vi "Main Page.vi"(8 "error in (no error)":errorcluster, 11 "Node Ptr":T1 format="%.0x") -> (0 "error out":errorcluster)   [LabVIEW 2015, in "Fuel Injector Analysis Addon System Explorer.lvlib"]
uses:
  Fuel Injector Analysis Addon System Explorer.lvlib
  <vilib>/NI Veristand/Custom Device API/Custom Device Item Ref.ctl
  <vilib>/NI/NI VeriStand Hardware Discovery/Types/Filter Type.ctl
  Shared/Constants.vi
  <vilib>/NI Veristand/Custom Device API/Set Item Property (String).vi
  <vilib>/NI Veristand/Custom Device API/Custom Device API.lvlib
  Shared/Fuel Injector Analysis Addon Shared.lvlib
  <vilib>/NI/NI VeriStand Hardware Discovery/NIVS Hardware Discovery.lvlib
panel:
  in  "RIO Browse":bool
  in  "SHDocVw.IWebBrowser":refnum<k7>(container)
  in  "Description":string
  in  "Sample Rate (Hz)":u32
  in  "RIO Device":string
  in  "Local Bitfile path":path
  in  "Header":cluster{"Section Name":string}={"Section Name"="Custom Device Item Settings"}
  in  "Name":string
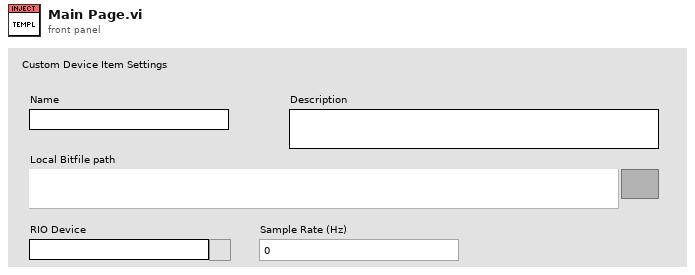
[diagram p1: front panel]
types:
  T1 = typedef "Custom Device API.lvlib/Custom Device Item Ref.ctl" = u64
  T2 = typedef "Custom Device API.lvlib/Custom Device Item Info.ctl" = cluster{"Name":string, "Is Channel":bool, "GUID":string, "Is Waveform":bool}
  T3 = typedef "Fuel Injector Analysis Addon Shared.lvlib/Main Settings.ctl" = cluster{"RIO Device Address":string, "Local bitfile path":path, "RT bitfile path":path, "Number of injectors":u16, "Sample rate (S/s)":u32}
  T4 = typedef "NIVS Hardware Discovery.lvlib/Filter Type.ctl" = enum16{"Device Category", "Product Name", "Ethernet", "XNET", "VISA", "FPGA", "EtherCAT Master", "DAQmx", "GPIB", "Serial"}
  T5 = enum16{"0", "1", "2", "3", "4", "5", "6", "7", "8"}
  T6 = typedef "Custom Device API.lvlib/Custom Device Commands.ctl" = enum16{"Default", "Item renamed", "Shutdown", "Dynamic button pressed"}
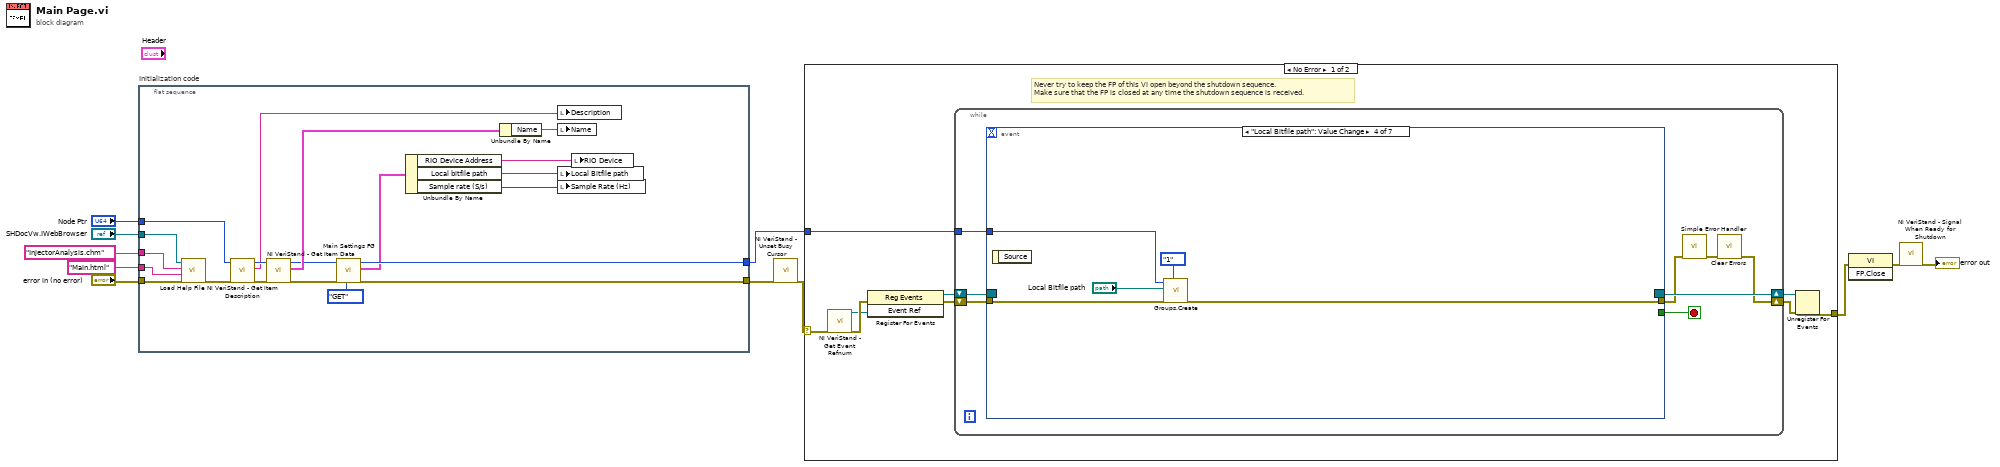
[diagram p0: block diagram]
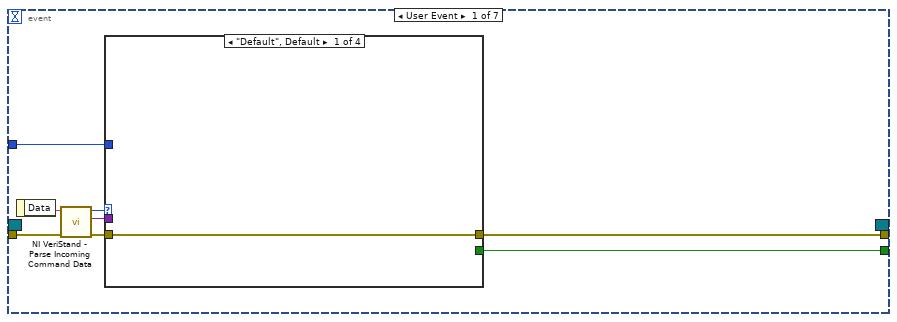
[diagram p2: hidden frame]
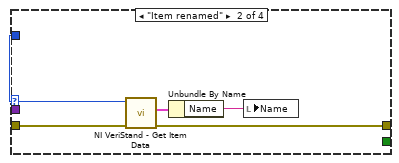
[diagram p3: hidden frame]
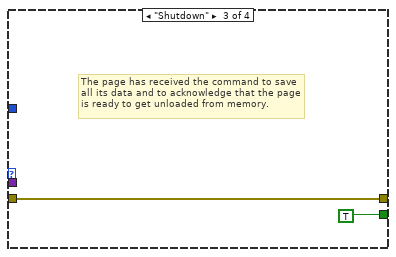
[diagram p4: hidden frame]
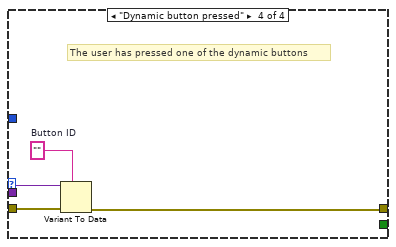
[diagram p5: hidden frame]
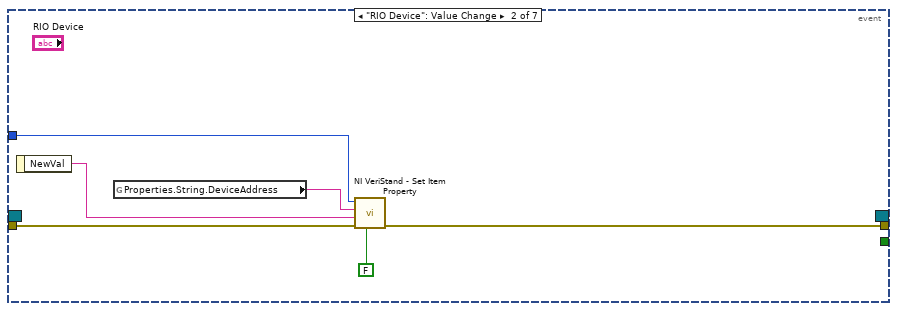
[diagram p6: hidden frame]
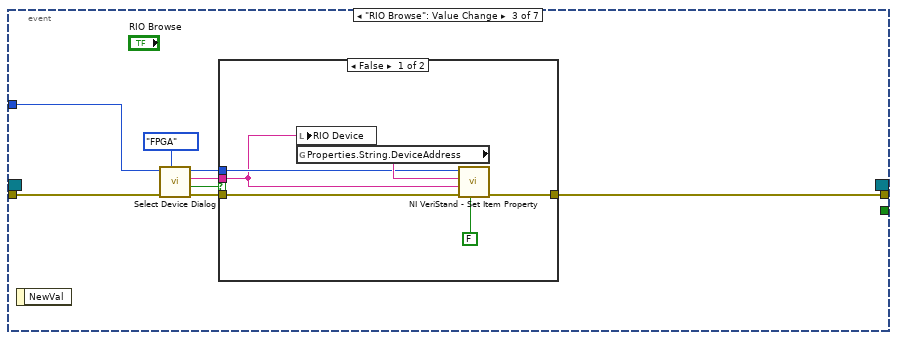
[diagram p7: hidden frame]
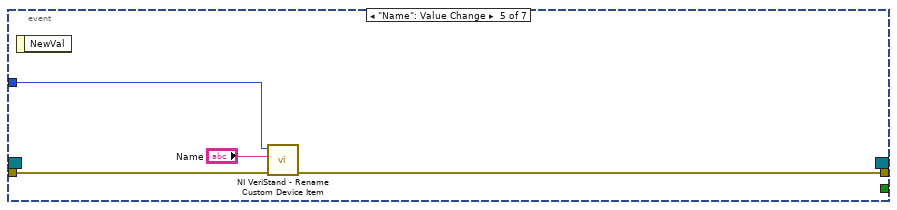
[diagram p9: hidden frame]
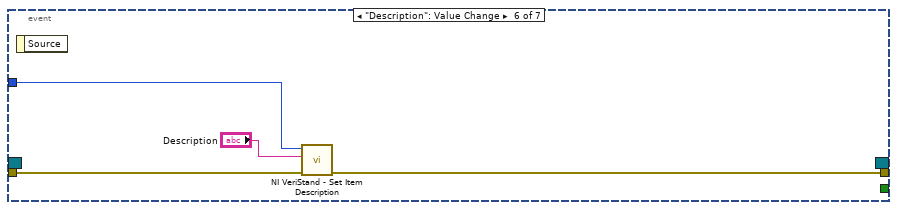
[diagram p10: hidden frame]
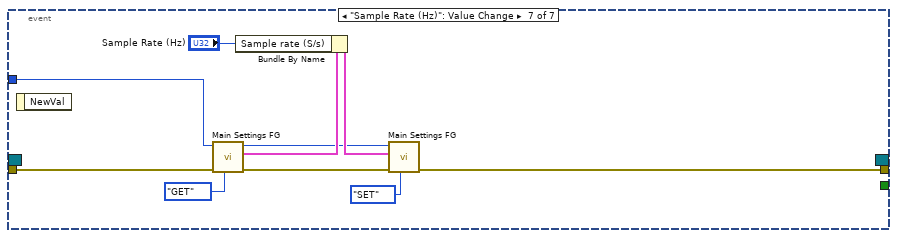
[diagram p11: hidden frame]
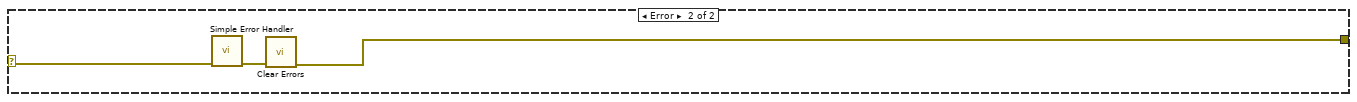
[diagram p12: hidden frame]
diagram:
  n1 = flat-sequence "Initialization code" {
    tunnel: "error in (no error)" -> [w16]
    tunnel: "Node Ptr" -> [w30]
    tunnel: [w12] -> w7
    tunnel: [w24] -> w4
    tunnel: "Main.html" ("HTML File") -> [w15]
    tunnel: "InjectorAnalysis.chm" ("Main CHM File") -> [w14]
    tunnel: "SHDocVw.IWebBrowser" -> [w13]
    frame #0 {
      n2 = call "Load Help File.vi"("error in (no error)"=w16, "HTML File"=w15, "Main CHM File"=w14, "SHDocVw.IWebBrowser2"=w13) -> ("error out"=w17:errorcluster)  [unwired: 7 in]
      n3 = call <vilib>:"NI VeriStand - Get Item Description.vi"("error in (no error)"=w17, "Item Ref in"=w30) -> ("error out"=w29:errorcluster, "Description"=w19:string, "Item Ref out"=w31:T1)  [unwired: 7 out]
      n4 = call <vilib>:"NI VeriStand - Get Item Data.vi"("error in (no error)"=w29, "Item Ref in"=w31) -> ("error out"=w26:errorcluster, "Item Info"=w28:T2, "Item Ref out"=w25:T1)  [unwired: 7 out]
      n5 = call "Main Settings FG.vi"("Action"=enum8{"GET", "SET"}."GET", "error in (no error)"=w26, "Item Ref"=w25) -> ("error out"=w12:errorcluster, "Main Settings out"=w22:T3, "Item Ref out"=w24:T1)  [unwired: 6 in]
      n6 = Unbundle By Name(w22) -> ("RIO Device Address"=w21:string, "Local bitfile path"=w20:path, "Sample rate (S/s)"=w18:u32)
      n7 = Unbundle By Name(w28) -> ("Name"=w27:string)
      n8 = local write "Description"(w19) -> ()
      n9 = local write "Name"(w27) -> ()
      n10 = local write "Local Bitfile path"(w20) -> ()
      n11 = local write "Sample Rate (Hz)"(w18) -> ()
      n12 = local write "RIO Device"(w21) -> ()
    }
  }
  n13 = call <vilib>:"NI VeriStand - Unset Busy Cursor.vi"("error in (no error)"=w7) -> ("error out"=w6:errorcluster)  [unwired: 10 out]
  n14 = case shown="No Error" w6 {
    selector: w6 -> [w32 w115]
    tunnel: [w37 w113] -> w11
    tunnel: w4 -> [w33 _]
    frame No Error {
      # "Never try to keep the FP of this VI open beyond the shutdown sequence.\nMake sure that the FP is closed at any time the shutdown sequence is received."
      n15 = call <vilib>:"NI VeriStand - Get Event Refnum.vi"("error in (no error)"=w32) -> ("error out"=w40:errorcluster, "Event Ref"=w36:refnum<user-event>)  [unwired: 9 out]
      n16 = register-events(error in=w40, w36) -> (reference out=w34:refnum<event-registration>, error out=w35:errorcluster)  [unwired: 1 in]
      n17 = while {
        tunnel: w33 -> [w44]
        shift-right: [w41] -> w38
        shift-left: w35 -> [w47]
        shift-right: [w48] -> w39
        shift-left: w34 -> [w46]
        stop <- w45 stop-if-true
        n18 = event shown="[3] \"Local Bitfile path\": Value Change" {
          selector: w46 -> [_ _ _ _ _ _ _]
          dyn-events: [_ _ _ _ _ _ _] -> w48
          timeout: _ -> [_ _ _ _ _ _ _]
          tunnel: w47 -> [w56 w74 w81 w92 w98 w102 w112]
          tunnel: [w52 _ _ _ _ _ _] -> w45
          tunnel: [w51 w70 w82 w94 w97 w99 w104] -> w43
          tunnel: w44 -> [w50 w71 w79 w91 w96 w101 w111]
          event User Event {
            n19 = event-data() -> ("Data"=w55:string)  [unwired: 1 out]
            n20 = call <vilib>:"NI VeriStand - Parse Incoming Command Data.vi"("error in (no error)"=w56, "Incoming data"=w55) -> ("error out"=w54:errorcluster, "Outgoing data"=w49:variant, "Action"=w53:T6)  [unwired: 7 out]
            n21 = case shown="\"Default\", Default" w53 {
              tunnel: w54 -> [w57 w62 w63 w68]
              tunnel: [_ _ TRUE _] -> w52
              tunnel: [w57 w59 w63 w65] -> w51
              tunnel: w50 -> [_ w61 _ _]
              tunnel: w49 -> [_ _ _ w67]
              frame "Default", Default {
              }
              frame "Item renamed" {
                n22 = call <vilib>:"NI VeriStand - Get Item Data.vi"("error in (no error)"=w62, "Item Ref in"=w61) -> ("error out"=w59:errorcluster, "Item Info"=w60:T2)  [unwired: 8 out]
                n23 = Unbundle By Name(w60) -> ("Name"=w58:string)
                n24 = local write "Name"(w58) -> ()
              }
              frame "Shutdown" {
                # "The page has received the command to save all its data and to acknowledge that the page is ready to get unloaded from memory."
              }
              frame "Dynamic button pressed" {
                w66 = ""  # Button ID
                # "The user has pressed one of the dynamic buttons"
                n25 = Variant To Data(error in=w68, type=w66, Variant=w67) -> (error out=w65:errorcluster)  [unwired: 1 out]
              }
            }
          }
          event "RIO Device": Value Change {
            n26 = event-data() -> ("NewVal"=w73:string)  [unwired: 1 out]
            n27 = global read "Constants.vi" "Properties.String.DeviceAddress"() -> (w72:string)
            n28 = call-poly <vilib>:"NI VeriStand - Set Item Property.vi"("Binary String (T)"=FALSE, "error in (no error)"=w74, "Value"=w73, "Property Name"=w72, "Item Ref in"=w71) -> ("error out"=w70:errorcluster)  [unwired: 4 in, 2 out]
          }
          event "RIO Browse": Value Change {
            n29 = event-data() -> ()  [unwired: 2 out]
            n30 = call <vilib>:"Select Device Dialog.vi"("Filter Type"=Filter_Type."FPGA", "error in (no error)"=w81, "Item Ref in"=w79) -> ("error out"=w80:errorcluster, "Cancelled?"=w77:bool, "Selected Alias"=w76:string, "Item Ref out"=w78:T1)  [unwired: 5 in]
            n31 = case shown="False" w77 {
              tunnel: w80 -> [w88 w89]
              tunnel: w78 -> [w86 _]
              tunnel: [w85 w89] -> w82
              tunnel: w76 -> [w83 _]
              frame False {
                n32 = local write "RIO Device"(w83) -> ()
                n33 = global read "Constants.vi" "Properties.String.DeviceAddress"() -> (w87:string)
                n34 = call-poly <vilib>:"NI VeriStand - Set Item Property.vi"("Binary String (T)"=FALSE, "error in (no error)"=w88, "Value"=w83, "Property Name"=w87, "Item Ref in"=w86) -> ("error out"=w85:errorcluster)  [unwired: 4 in, 2 out]
              }
              frame True {
              }
            }
          }
          event "Local Bitfile path": Value Change {
            n35 = event-data() -> ()  [unwired: 2 out]
            n36 = call "Groups.Create.vi"("Max Shots"=T5."1", "error in (no error)"=w92, "NewVal"="Local Bitfile path", "Item Ref in"=w91) -> ("error out"=w94:errorcluster)  [unwired: 6 in, 1 out]
          }
          event "Name": Value Change {
            n37 = event-data() -> ()  [unwired: 2 out]
            n38 = call <vilib>:"NI VeriStand - Rename Custom Device Item.vi"("error in (no error)"=w98, "New Name"="Name", "Item Ref in"=w96) -> ("error out"=w97:errorcluster)  [unwired: 1 in, 7 out]
          }
          event "Description": Value Change {
            n39 = event-data() -> ()  [unwired: 2 out]
            n40 = call <vilib>:"NI VeriStand - Set Item Description.vi"("error in (no error)"=w102, "Description"="Description", "Item Ref in"=w101) -> ("error out"=w99:errorcluster)  [unwired: 6 in, 2 out]
          }
          event "Sample Rate (Hz)": Value Change {
            n41 = event-data() -> ()  [unwired: 2 out]
            n42 = call "Main Settings FG.vi"("Action"=enum8{"GET", "SET"}."GET", "error in (no error)"=w112, "Item Ref"=w111) -> ("error out"=w109:errorcluster, "Main Settings out"=w108:T3, "Item Ref out"=w105:T1)  [unwired: 6 in]
            n43 = Bundle By Name(cluster=w108, "Sample rate (S/s)"="Sample Rate (Hz)") -> (w107:T3)
            n44 = call "Main Settings FG.vi"("Action"=enum8{"GET", "SET"}."SET", "error in (no error)"=w109, "Main Settings"=w107, "Item Ref"=w105) -> ("error out"=w104:errorcluster)  [unwired: 5 in, 2 out]
          }
        }
        n45 = call <vilib>:"Simple Error Handler.vi"("error in (no error)"=w43) -> ("error out"=w42:errorcluster)  [unwired: 1 in, 7 out]
        n46 = call <vilib>:"Clear Errors.vi"("error in (no error)"=w42) -> ("error out"=w41:errorcluster)  [unwired: 1 in, 5 out]
      }
      n47 = Unregister For Events(event registration refnum=w39, error in=w38) -> (error out=w37:errorcluster)
    }
    frame Error {
      n48 = call <vilib>:"Simple Error Handler.vi"("error in (no error)"=w115) -> ("error out"=w114:errorcluster)  [unwired: 1 in, 7 out]
      n49 = call <vilib>:"Clear Errors.vi"("error in (no error)"=w114) -> ("error out"=w113:errorcluster)  [unwired: 1 in, 5 out]
    }
  }
  n50 = invoke class="VI" method="FP.Close"(error in=w11) -> (error out=w10:errorcluster)  [unwired: 2 in, 2 out]
  n51 = call <vilib>:"NI VeriStand - Signal When Ready for Shutdown.vi"("error in (no error)"=w10) -> ("error out"=→"error out":errorcluster)  [unwired: 10 out]
